vi "Add Subscriber.vi"(8 "error in (no error)":errorcluster, 9 "Subscription Object":refnum<class>, 10 "Subscriber Enqueuer":refnum<class "Message Enqueuer.lvclass">, 11 "Subsciptions in":T1[](array[typedef])) -> (0 "error out":errorcluster, 3 "Subsciptions out":T1[](array[typedef]))   [LabVIEW 2020, in "Publisher.lvlib" / "Publisher.lvclass"]
doc: "Add the 'Subscriber Enqueuer' to the 'Subscriptions' using the 'Subscription string'."
uses:
  Publisher.lvclass
  PPL/HDH.Actor Framework.Core.Actor.lvlibp/1abvi3w/vi.lib/ActorFramework/Message Enqueuer/Message Enqueuer.lvclass
  Controls/Ctl_Subscription Element.ctl
  9bfa7042-f496-41a0-bdb3-f05adf9a1a12.vi
  PPL/HDH.Actor Framework.Core.Utility.lvlibp
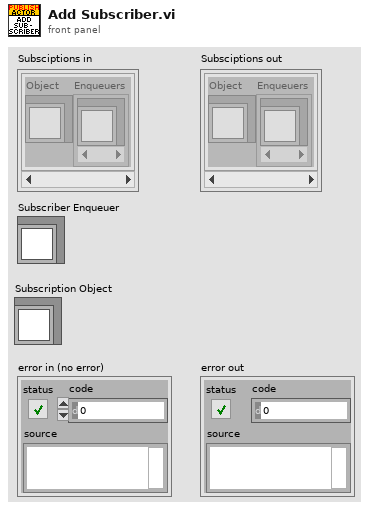
[diagram p1: front panel]
types:
  T1 = typedef "Publisher.lvlib/Publisher.lvclass/Ctl_Subscription Element.ctl" = cluster{"Object":refnum<class>, "Enqueuers":refnum<class "Message Enqueuer.lvclass">[]}
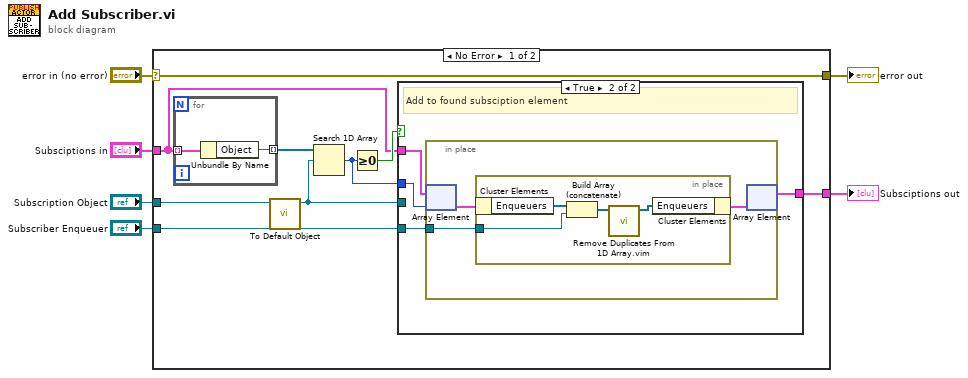
[diagram p0: block diagram]
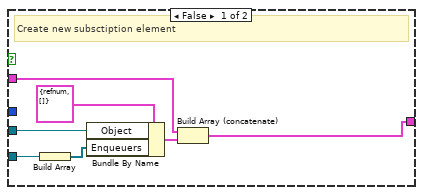
[diagram p2: hidden frame]
diagram:
  n1 = case shown="No Error" "error in (no error)" {
    selector: "error in (no error)" -> [w7 w37]
    tunnel: "Subscription Object" -> [w15 _]
    tunnel: "Subsciptions in" -> [w12 w36]
    tunnel: "Subscriber Enqueuer" -> [w10 _]
    tunnel: [w9 w36] -> w3
    tunnel: [w7 w37] -> w2
    frame No Error {
      n2 = for {
        tunnel: w12 -> [w35] mode=indexing
        tunnel: [w34] -> w14 mode=indexing
        n3 = Unbundle By Name(w35) -> ("Object"=w34:refnum<class>)
      }
      n4 = call "To Default Object.vi"("Object in"=w15) -> ("Default out"=w11:refnum<class>)  [unwired: 10 in]
      n5 = Search 1D Array(1D array=w14, element=w11) -> (index of element=w8:i32)  [unwired: 1 in]
      n6 = Greater Or Equal To 0?(x=w8) -> (x >= 0?=w13:bool)
      n7 = case shown="True" w13 {
        tunnel: w12 -> [w19 w26]
        tunnel: w11 -> [w22 _]
        tunnel: w10 -> [w21 w24]
        tunnel: [w18 w25] -> w9
        tunnel: w8 -> [_ w23]
        frame False {
          # "Create new subsctiption element"
          n8 = Build Array(w21) -> (w20:refnum<class "Message Enqueuer.lvclass">[])
          n9 = Bundle By Name(cluster=T1 {"Object"=refnum, "Enqueuers"=[]} ("Subsciption element"), "Object"=w22, "Enqueuers"=w20) -> (w16:T1)
          n10 = Build Array (concatenate)(w19, w16) -> (w18:T1[])
        }
        frame True {
          # "Add to found subsciption element"
          n11 = in-place {
            in-place-border: w24 -> [w28]
            n12 = in-place-array #1(w26, w23) -> (w29:T1)
            n13 = in-place {
              in-place-border: w28 -> [w32]
              n14 = in-place-cluster #2(w29) -> ("Enqueuers"=w33:refnum<class "Message Enqueuer.lvclass">[])
              n15 = Build Array (concatenate)(w33, w32) -> (w31:refnum<class "Message Enqueuer.lvclass">[])
              n16 = call "Remove Duplicates From 1D Array.vim"("array"=w31) -> ("array with duplicates removed"=w30:refnum<class "Message Enqueuer.lvclass">[])  [unwired: 10 in]
              n17 = in-place-cluster #2("Enqueuers"=w30) -> (w27:T1)
            }
            n18 = in-place-array #1(w27) -> (w25:T1[])  [unwired: 1 out]
          }
        }
      }
    }
    frame Error {
    }
  }
  "error out" <- w2
  "Subsciptions out" <- w3
